vi "DeltaE(2000).vi"(1 "L*a*b Colors":T1) -> (0 "Delta E":dbl)   [LabVIEW 2013]
panel:
  out "D L'":dbl
  out "D C'":dbl
  out "Rt":dbl
  out "Sc":dbl
  out "Sh":dbl
  out "Sl":dbl
  out "DH":dbl
  out "H'":dbl
  out "T":dbl
  out "D h'":dbl
  out "L'_":dbl
  out "C'_":dbl
  out "C2'":dbl
  out "C1'":dbl
  out "a2'":dbl
  out "a1'":dbl
  out "G":dbl
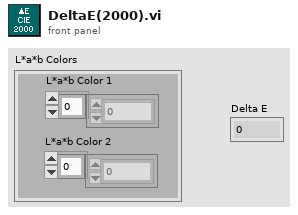
[diagram p1: front panel]
types:
  T1 = cluster{"L*a*b Color 1":dbl[], "L*a*b Color 2":dbl[]}
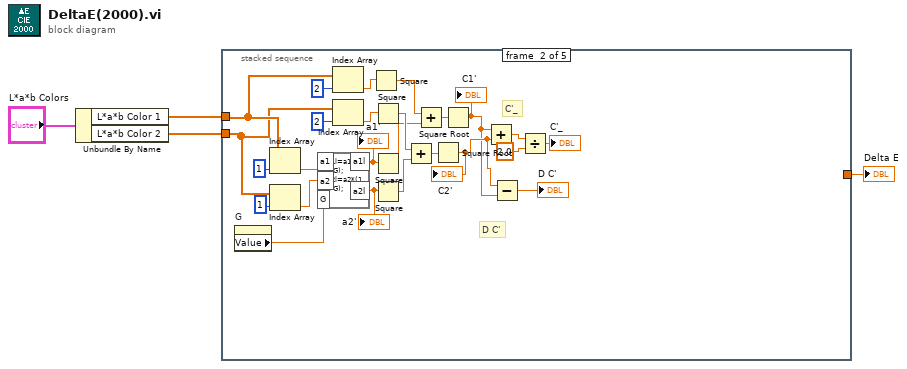
[diagram p0: block diagram]
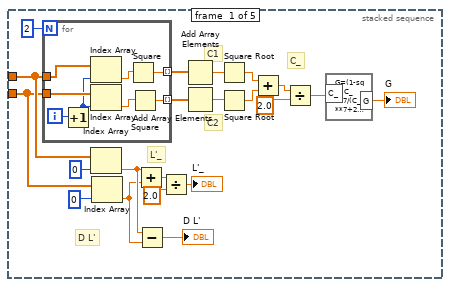
[diagram p2: hidden frame]
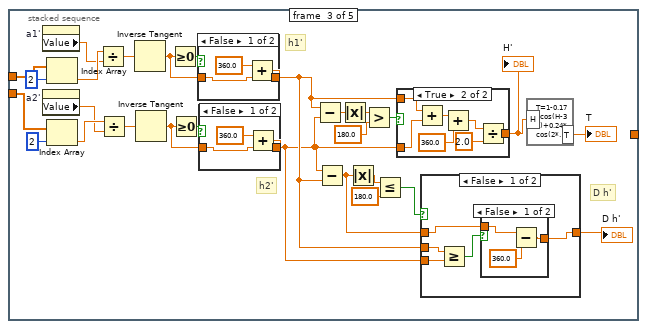
[diagram p3: hidden frame]
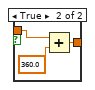
[diagram p4: hidden frame]
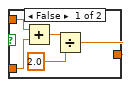
[diagram p6: hidden frame]
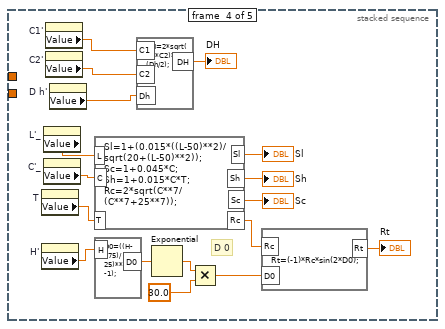
[diagram p9: hidden frame]
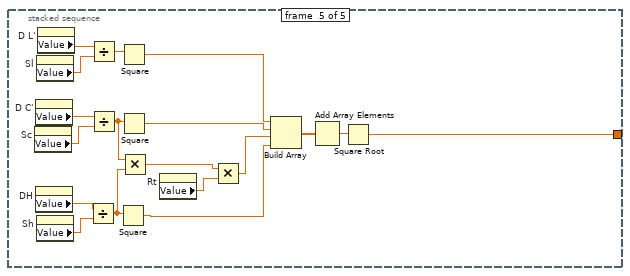
[diagram p10: hidden frame]
diagram:
  n1 = Unbundle By Name("L*a*b Colors") -> ("L*a*b Color 1"=w3:dbl[], "L*a*b Color 2"=w2:dbl[])
  n2 = stacked-sequence {
    tunnel: w3 -> [w16 w51 w85 _ _]
    tunnel: w2 -> [w15 w50 w82 _ _]
    tunnel: [_ _ _ _ w135] -> w1
    frame #0 {
      # "D L'"
      # "L'_"
      # "C_"
      # "C2"
      # "C1"
      n3 = for {
        N: 2 -> [_]
        tunnel: w16 -> [w32]
        tunnel: w15 -> [w31]
        tunnel: [w27] -> w24 mode=indexing
        tunnel: [w26] -> w23 mode=indexing
        i -> [w33]
        n4 = Increment(x=w33) -> (x+1=w30:i32)
        n5 = Index Array(array=w32, index=w30) -> (element=w29:dbl)
        n6 = Index Array(array=w31, index=w30) -> (element=w28:dbl)
        n7 = Square(x=w29) -> (x^2=w27:dbl)
        n8 = Square(x=w28) -> (x^2=w26:dbl)
      }
      n9 = Index Array(array=w16, index=0) -> (element=w10:dbl)
      n10 = Index Array(array=w15, index=0) -> (element=w9:dbl)
      n11 = Add(x=w10, y=w9) -> (x+y=w12:dbl)
      n12 = Subtract(x=w10, y=w9) -> (x-y=→"D L'":dbl)
      n13 = Divide(x=w12, y=2.0) -> (x/y=→"L'_":dbl)
      n14 = Add Array Elements(numeric array=w24) -> (sum=w22:dbl)
      n15 = Add Array Elements(numeric array=w23) -> (sum=w21:dbl)
      n16 = Square Root(x=w22) -> (sqrt(x)=w20:dbl)
      n17 = Square Root(x=w21) -> (sqrt(x)=w19:dbl)
      n18 = Add(x=w20, y=w19) -> (x+y=w18:dbl)
      n19 = Divide(x=w18, y=2.0) -> (x/y=w8:dbl)
      n20 = formula code="G=(1-sqrt(C_**7/(C_**7+25**7)))/2;"("C_"=w8) -> ("G"=→"G":dbl)
    }
    frame #1 {
      # "D C'"
      # "C'_"
      n21 = property on="G" class="DigNum (strict)"() -> ("Value"=w54:dbl)  [unwired: 2 in, 2 out]
      n22 = Index Array(array=w51, index=1) -> (element=w56:dbl)
      n23 = Index Array(array=w50, index=1) -> (element=w55:dbl)
      n24 = formula code="a1l=a1*(1+G);\na2l=a2*(1+G);"("a1"=w56, "a2"=w55, "G"=w54) -> ("a1l"=w52:dbl, "a2l"=w53:dbl)
      "a1'" <- w52
      "a2'" <- w53
      n25 = Index Array(array=w51, index=2) -> (element=w47:dbl)
      n26 = Index Array(array=w50, index=2) -> (element=w46:dbl)
      n27 = Square(x=w47) -> (x^2=w43:dbl)
      n28 = Square(x=w46) -> (x^2=w45:dbl)
      n29 = Square(x=w52) -> (x^2=w42:dbl)
      n30 = Square(x=w53) -> (x^2=w44:dbl)
      n31 = Add(x=w45, y=w44) -> (x+y=w41:dbl)
      n32 = Add(x=w43, y=w42) -> (x+y=w40:dbl)
      n33 = Square Root(x=w41) -> (sqrt(x)=w37:dbl)
      "C2'" <- w37
      n34 = Square Root(x=w40) -> (sqrt(x)=w36:dbl)
      "C1'" <- w36
      n35 = Add(x=w36, y=w37) -> (x+y=w39:dbl)
      n36 = Subtract(x=w37, y=w36) -> (x-y=→"D C'":dbl)
      n37 = Divide(x=w39, y=2.0) -> (x/y=→"C'_":dbl)
    }
    frame #2 {
      # "D h'"
      # "h2'"
      # "h1'"
      n38 = property on="a1'" class="DigNum (strict)"() -> ("Value"=w80:dbl)  [unwired: 2 in, 2 out]
      n39 = property on="a2'" class="DigNum (strict)"() -> ("Value"=w72:dbl)  [unwired: 2 in, 2 out]
      n40 = Index Array(array=w85, index=2) -> (element=w81:dbl)
      n41 = Index Array(array=w82, index=2) -> (element=w73:dbl)
      n42 = Divide(x=w81, y=w80) -> (x/y=w79:dbl)
      n43 = Divide(x=w73, y=w72) -> (x/y=w76:dbl)
      n44 = Inverse Tangent(1:w79) -> (0:w77:dbl)
      n45 = Inverse Tangent(1:w76) -> (0:w74:dbl)
      n46 = Greater Or Equal To 0?(x=w77) -> (x >= 0?=w78:bool)
      n47 = Greater Or Equal To 0?(x=w74) -> (x >= 0?=w75:bool)
      n48 = case shown="False" w78 {
        tunnel: w77 -> [w115 w117]
        tunnel: [w114 w117] -> w63
        frame False {
          n49 = Add(x=360.0, y=w115) -> (x+y=w114:dbl)
        }
        frame True {
        }
      }
      n50 = case shown="False" w75 {
        tunnel: w74 -> [w111 w113]
        tunnel: [w110 w113] -> w62
        frame False {
          n51 = Add(x=360.0, y=w111) -> (x+y=w110:dbl)
        }
        frame True {
        }
      }
      n52 = Subtract(x=w63, y=w62) -> (x-y=w71:dbl)
      n53 = Subtract(x=w62, y=w63) -> (x-y=w64:dbl)
      n54 = Absolute Value(x=w71) -> (abs(x)=w70:dbl)
      n55 = Absolute Value(x=w64) -> (abs(x)=w67:dbl)
      n56 = Greater?(x=w70, y=180.0) -> (0:w68:bool)
      n57 = Less Or Equal?(x=w67, y=180.0) -> (x <= y?=w65:bool)
      n58 = case shown="True" w68 {
        tunnel: w63 -> [w102 w109]
        tunnel: w62 -> [w101 w108]
        tunnel: [w98 w103] -> w61
        frame False {
          n59 = Add(x=w102, y=w101) -> (x+y=w100:dbl)
          n60 = Divide(x=w100, y=2.0) -> (x/y=w98:dbl)
        }
        frame True {
          n61 = Add(x=w109, y=w108) -> (x+y=w107:dbl)
          n62 = Add(x=w107, y=360.0) -> (x+y=w105:dbl)
          n63 = Divide(x=w105, y=2.0) -> (x/y=w103:dbl)
        }
      }
      "H'" <- w61
      n64 = case shown="False" w65 {
        tunnel: w64 -> [w87 w97]
        tunnel: [w86 w97] -> w60
        tunnel: w63 -> [w89 _]
        tunnel: w62 -> [w90 _]
        frame False {
          n65 = Greater Or Equal?(x=w89, y=w90) -> (x >= y?=w88:bool)
          n66 = case shown="False" w88 {
            tunnel: w87 -> [w93 w96]
            tunnel: [w91 w95] -> w86
            frame False {
              n67 = Subtract(x=w93, y=360.0) -> (x-y=w91:dbl)
            }
            frame True {
              n68 = Add(x=w96, y=360.0) -> (x+y=w95:dbl)
            }
          }
        }
        frame True {
        }
      }
      "D h'" <- w60
      n69 = formula code="T=1-0.17*cos(H-30)+0.24*cos(2*H)+0.32*cos(3*H+6)-0.2*cos(4*H-63);"("H"=w61) -> ("T"=→"T":dbl)
    }
    frame #3 {
      # "D 0"
      n70 = property on="T" class="DigNum (strict)"() -> ("Value"=w129:dbl)  [unwired: 2 in, 2 out]
      n71 = property on="H'" class="DigNum (strict)"() -> ("Value"=w128:dbl)  [unwired: 2 in, 2 out]
      n72 = property on="L'_" class="DigNum (strict)"() -> ("Value"=w131:dbl)  [unwired: 2 in, 2 out]
      n73 = property on="C'_" class="DigNum (strict)"() -> ("Value"=w130:dbl)  [unwired: 2 in, 2 out]
      n74 = property on="C1'" class="DigNum (strict)"() -> ("Value"=w134:dbl)  [unwired: 2 in, 2 out]
      n75 = property on="C2'" class="DigNum (strict)"() -> ("Value"=w133:dbl)  [unwired: 2 in, 2 out]
      n76 = property on="D h'" class="DigNum (strict)"() -> ("Value"=w132:dbl)  [unwired: 2 in, 2 out]
      n77 = formula code="Sl=1+(0.015*((L-50)**2)/sqrt(20+(L-50)**2));\nSc=1+0.045*C;\nSh=1+0.015*C*T;\nRc=2*sqrt(C**7/(C**7+25**7));"("L"=w131, "C"=w130, "T"=w129) -> ("Sl"=→"Sl":dbl, "Sh"=→"Sh":dbl, "Sc"=→"Sc":dbl, "Rc"=w120:dbl)
      n78 = formula code="D0=((H-275)/25)**2*(-1);"("H"=w128) -> ("D0"=w127:dbl)
      n79 = formula code="DH=2*sqrt(C1*C2)*sin(Dh/2);"("C1"=w134, "C2"=w133, "Dh"=w132) -> ("DH"=→"DH":dbl)
      n80 = Exponential(1:w127) -> (0:w126:dbl)
      n81 = Multiply(x=w126, y=30.0) -> (x*y=w119:dbl)
      n82 = formula code="Rt=(-1)*Rc*sin(2*D0);"("Rc"=w120, "D0"=w119) -> ("Rt"=→"Rt":dbl)
    }
    frame #4 {
      n83 = property on="Sc" class="DigNum (strict)"() -> ("Value"=w149:dbl)  [unwired: 2 in, 2 out]
      n84 = property on="D C'" class="DigNum (strict)"() -> ("Value"=w150:dbl)  [unwired: 2 in, 2 out]
      n85 = property on="DH" class="DigNum (strict)"() -> ("Value"=w148:dbl)  [unwired: 2 in, 2 out]
      n86 = property on="Sl" class="DigNum (strict)"() -> ("Value"=w151:dbl)  [unwired: 2 in, 2 out]
      n87 = property on="Sh" class="DigNum (strict)"() -> ("Value"=w147:dbl)  [unwired: 2 in, 2 out]
      n88 = property on="D L'" class="DigNum (strict)"() -> ("Value"=w152:dbl)  [unwired: 2 in, 2 out]
      n89 = Divide(x=w148, y=w147) -> (x/y=w144:dbl)
      n90 = Divide(x=w152, y=w151) -> (x/y=w146:dbl)
      n91 = Divide(x=w150, y=w149) -> (x/y=w145:dbl)
      n92 = Square(x=w144) -> (x^2=w141:dbl)
      n93 = Square(x=w146) -> (x^2=w138:dbl)
      n94 = Square(x=w145) -> (x^2=w139:dbl)
      n95 = Multiply(x=w145, y=w144) -> (x*y=w142:dbl)
      n96 = property on="Rt" class="DigNum (strict)"() -> ("Value"=w143:dbl)  [unwired: 2 in, 2 out]
      n97 = Multiply(x=w142, y=w143) -> (x*y=w140:dbl)
      n98 = Build Array(w138, w139, w140, w141) -> (w137:dbl[])
      n99 = Add Array Elements(numeric array=w137) -> (sum=w136:dbl)
      n100 = Square Root(x=w136) -> (sqrt(x)=w135:dbl)
    }
  }
  "Delta E" <- w1
